vi "Point_Set_Attribute.vi"(6 "Value":string, 8 "Error In":errorcluster, 9 "Attribute":string, 10 "Tag":string, 11 "Map":T1) -> (0 "Error Out":errorcluster, 3 "Map Out":T1)   [LabVIEW 2017, in "PointValueMap.lvlib"]
doc: "Sets a named attribute and value on a map point."
uses:
  <vilib>/addons/PointValueMap/PointValueMap.lvlib
  <vilib>/addons/PointValueMap/controls/PointMap.ctl
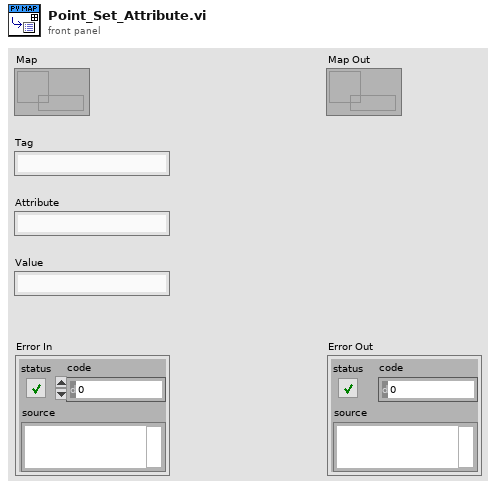
[diagram p1: front panel]
types:
  T1 = typedef "PointValueMap.lvlib/PointMap.ctl" = refnum<data-value>
  T2 = typedef "PointValueMap.lvlib/Point.ctl" = cluster{"Datatype":T3, "Timestamp":timestamp, "Value":variant, "Valid":bool}
  T3 = typedef "PointValueMap.lvlib/DataTypes.ctl" = enum16{"single", "double", "i32", "string", "variant"}
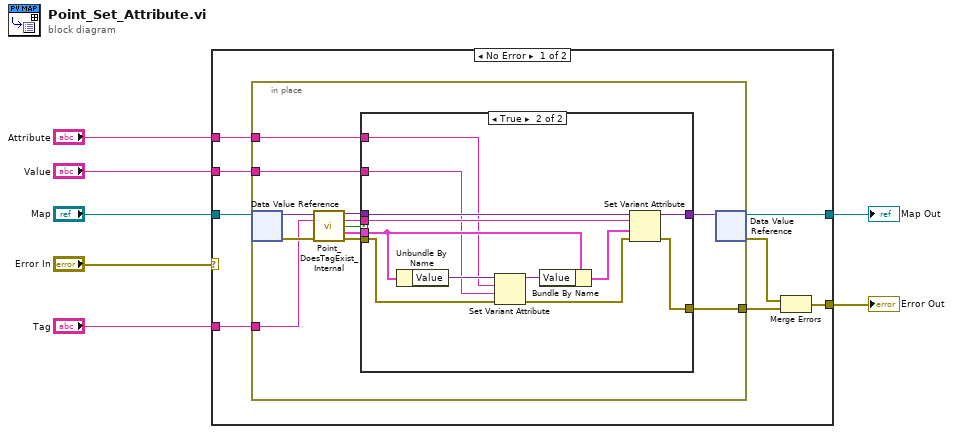
[diagram p0: block diagram]
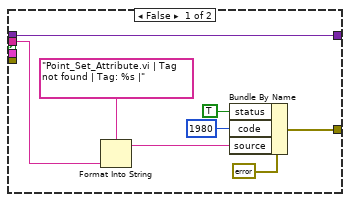
[diagram p2: hidden frame]
diagram:
  n1 = case shown="No Error" "Error In" {
    selector: "Error In" -> [_ w49]
    tunnel: "Map" -> [w15 w48]
    tunnel: "Tag" -> [w14 _]
    tunnel: [w11 w49] -> w6
    tunnel: "Attribute" -> [w10 _]
    tunnel: "Value" -> [w9 _]
    tunnel: [w8 w48] -> w1
    frame No Error {
      n2 = in-place {
        in-place-border: w14 -> [w18]
        in-place-border: [w26] -> w12
        in-place-border: w10 -> [w25]
        in-place-border: w9 -> [w24]
        n3 = in-place-dvr #1(w15) -> (w23:variant, w21:errorcluster)
        n4 = call <vilib>:"Point_DoesTagExist_Internal.vi"("Map"=w23, "Tag"=w18, "Error In"=w21) -> ("Map Out"=w22:variant, "Tag Out"=w16:string, "Tag Exists"=w19:bool, "Point"=w17:T2, "Error Out"=w20:errorcluster)  [unwired: 7 in, 1 out]
        n5 = case shown="True" w19 {
          tunnel: [w29 w47] -> w27
          tunnel: [w30 w46] -> w26
          tunnel: w25 -> [_ w39]
          tunnel: w24 -> [_ w38]
          tunnel: w22 -> [w29 w45]
          tunnel: w20 -> [_ w37]
          tunnel: w17 -> [_ w44]
          tunnel: w16 -> [w28 w42]
          frame False {
            n6 = Format Into String(format string="Point_Set_Attribute.vi | Tag not found | Tag: %s |" ("source"), w28) -> (resulting string=w32:string)  [unwired: 2 in, 1 out]
            n7 = Bundle By Name(cluster=errorcluster {"status"=FALSE, "code"=0, "source"=""} ("Error Out"), "status"=TRUE, "code"=1980, "source"=w32) -> (w30:errorcluster)
          }
          frame True {
            n8 = Unbundle By Name(w44) -> ("Value"=w41:variant)
            n9 = Set Variant Attribute(Variant=w41, name=w39, value=w38, error in=w37) -> (Variant out=w40:variant, error out=w36:errorcluster)  [unwired: 1 out]
            n10 = Bundle By Name(cluster=w44, "Value"=w40) -> (w43:T2)
            n11 = Set Variant Attribute(Variant=w45, name=w42, value=w43, error in=w36) -> (Variant out=w47:variant, error out=w46:errorcluster)  [unwired: 1 out]
          }
        }
        n12 = in-place-dvr #1(w27) -> (w8:T1, w13:errorcluster)
      }
      n13 = Merge Errors(w13, w12) -> (w11:errorcluster)
    }
    frame Error {
    }
  }
  "Error Out" <- w6
  "Map Out" <- w1
